vi "numCmd_Recv_Generic.vi"(7 "Command Name":string, 11 "Initial Value":variant) -> (0 "error out":errorcluster, 2 "Changed":bool, 3 "Newest Value":variant)   [LabVIEW 2019, in "Trajectory_Library.lvlib"]
uses:
  Trajectory_Library.lvlib
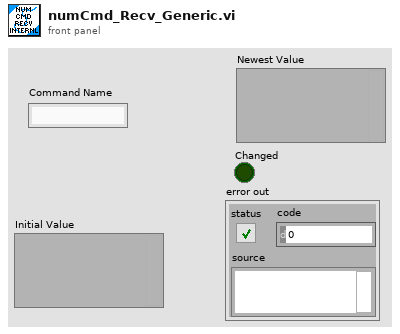
[diagram p1: front panel]
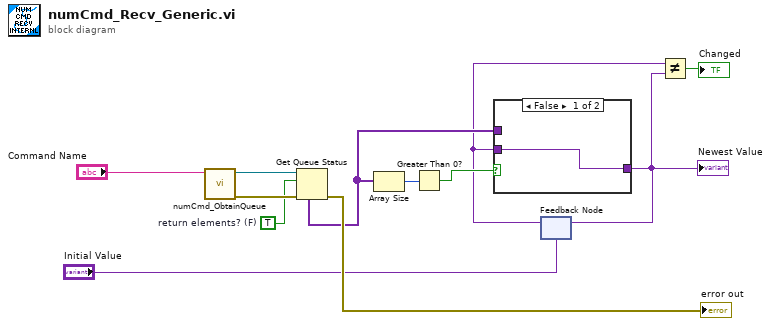
[diagram p0: block diagram]
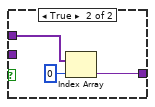
[diagram p2: hidden frame]
diagram:
  w1 = TRUE  # return elements? (F)
  n1 = call "numCmd_ObtainQueue.vi"("Command Name"="Command Name") -> ("error out"=w10:errorcluster, "queue out"=w11:refnum<queue>)  [unwired: 9 in]
  n2 = Get Queue Status(queue=w11, return elements? (F)=w1, error in (no error)=w10) -> (error out=→"error out":errorcluster, elements=w5:variant[])  [unwired: 6 out]
  n3 = Array Size(array=w5) -> (size(s)=w9:i32)
  n4 = Greater Than 0?(x=w9) -> (x > 0?=w6:bool)
  n5 = feedback #1("Initial Value") -> (w2:variant)
  n6 = case shown="False" w6 {
    tunnel: w5 -> [_ w16]
    tunnel: [w13 w14] -> w3
    tunnel: w2 -> [w13 _]
    frame False {
    }
    frame True {
      n7 = Index Array(array=w16, index=0) -> (element=w14:variant)
    }
  }
  "Newest Value" <- w3
  n8 = feedback-in #1(w3) -> ()
  n9 = Not Equal?(x=w2, y=w3) -> (x != y?=→"Changed":bool)
